vi "Main.vi"() -> ()   [LabVIEW 2018]
doc: "This VI simulates the acquisition of temperature, graphs the temperature, and notifies the user if the temperature is over the limit.\n\nThis VI is an exercise in the LabVIEW Basics II course and is used to experience property nodes."
panel:
  in  "Switch":bool
  in  "?":bool
  in  "Points to Acquire 8":i32=75 min=20 max=500
  in  "Points to Acquire 7":i32=75 min=20 max=500
  in  "Points to Acquire 6":i32=75 min=20 max=500
  in  "?":bool
  out "Remaining Time in Seconds":dbl
  in  "?":T1(tab)
  out "Temperature 2":T2(graph)
  out "5% Humidity":bool
  out "Temperature 9":T2(graph)
  out "5% Humidity":bool
  out "Temperature 10":T2(graph)
  out "5% Humidity":bool
  out "Temperature 11":T2(graph)
  out "5% Humidity":bool
  out "Weight Scale":dbl(knob) scale=0.0..10.0 scale format="%^#_6g"
  out "Weight Text Display":string
  in  "?":T3(tab)
  out "Temperature 3":T4(graph)
  out "7% Humidity":bool
  out "Temperature 6":T4(graph)
  out "7% Humidity":bool
  out "Temperature 7":T4(graph)
  out "7% Humidity":bool
  out "Temperature 8":T4(graph)
  out "7% Humidity":bool
  in  "Insert Cashew Nut Humidity Here":path
  in  "Insert Cashew Nut Weight":path
  in  "Heating Capacity":u32=400 min=50 max=2000 step=50
  out "Overload":bool
  in  "Points to Acquire 2":i32=75 min=20 max=500
  # "Drying Device"
  # "Roasting Device"
  # "Cashew Parameters"
  # "Device Parameters"
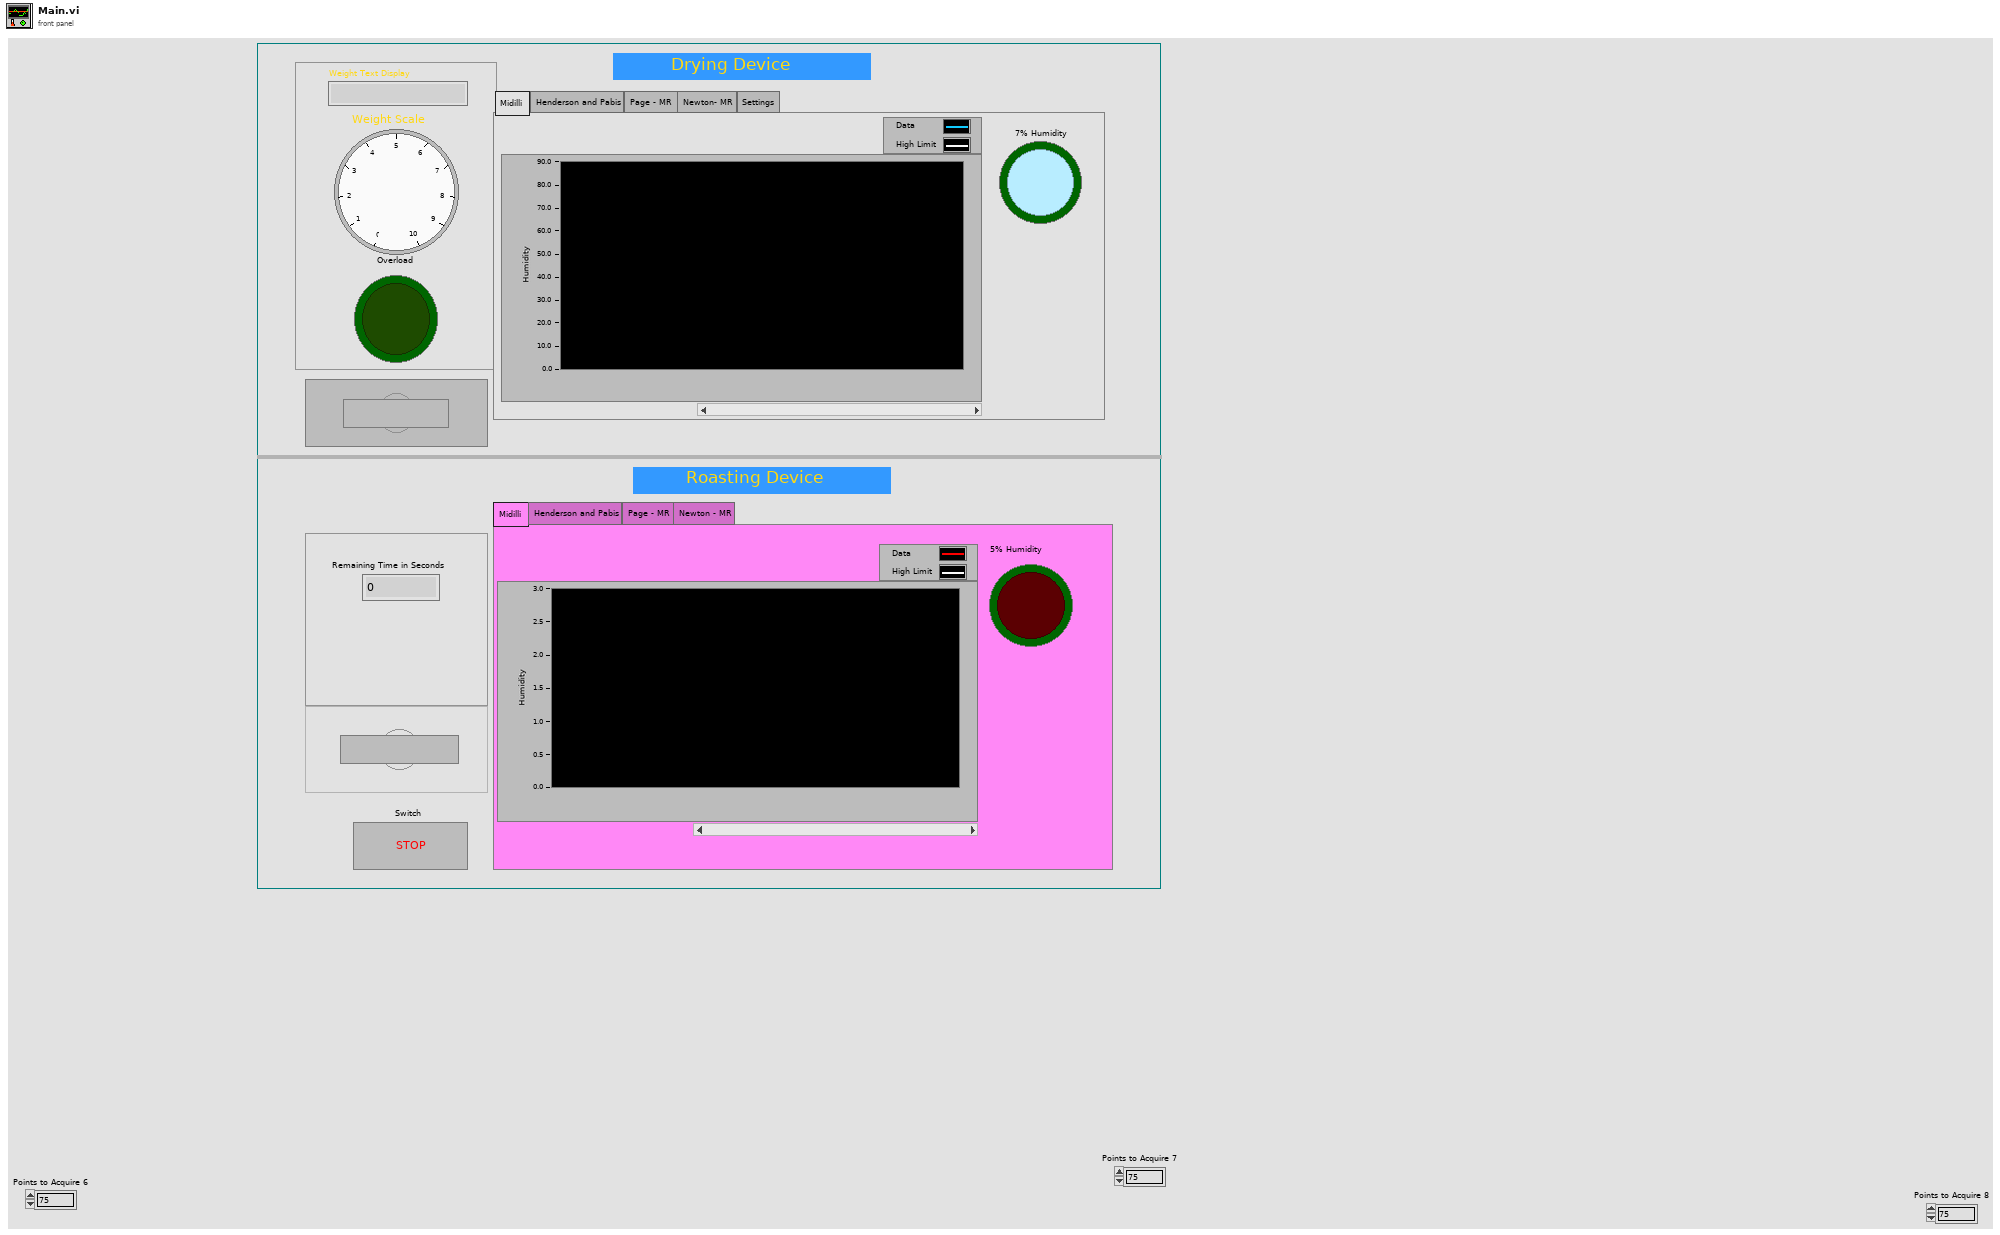
[diagram p1: front panel]
types:
  T1 = enum32{"Midilli", "Henderson and Pabis", "Page - MR", "Newton - MR"}
  T2 = cluster{"Temperature":dbl, "Temp High Limit 2":dbl}
  T3 = enum32{"Midilli", "Henderson and Pabis", "Page - MR ", "Newton- MR", "Settings"}
  T4 = cluster{"Humidity  High Limit":dbl, "Cashew Humidity":dbl}
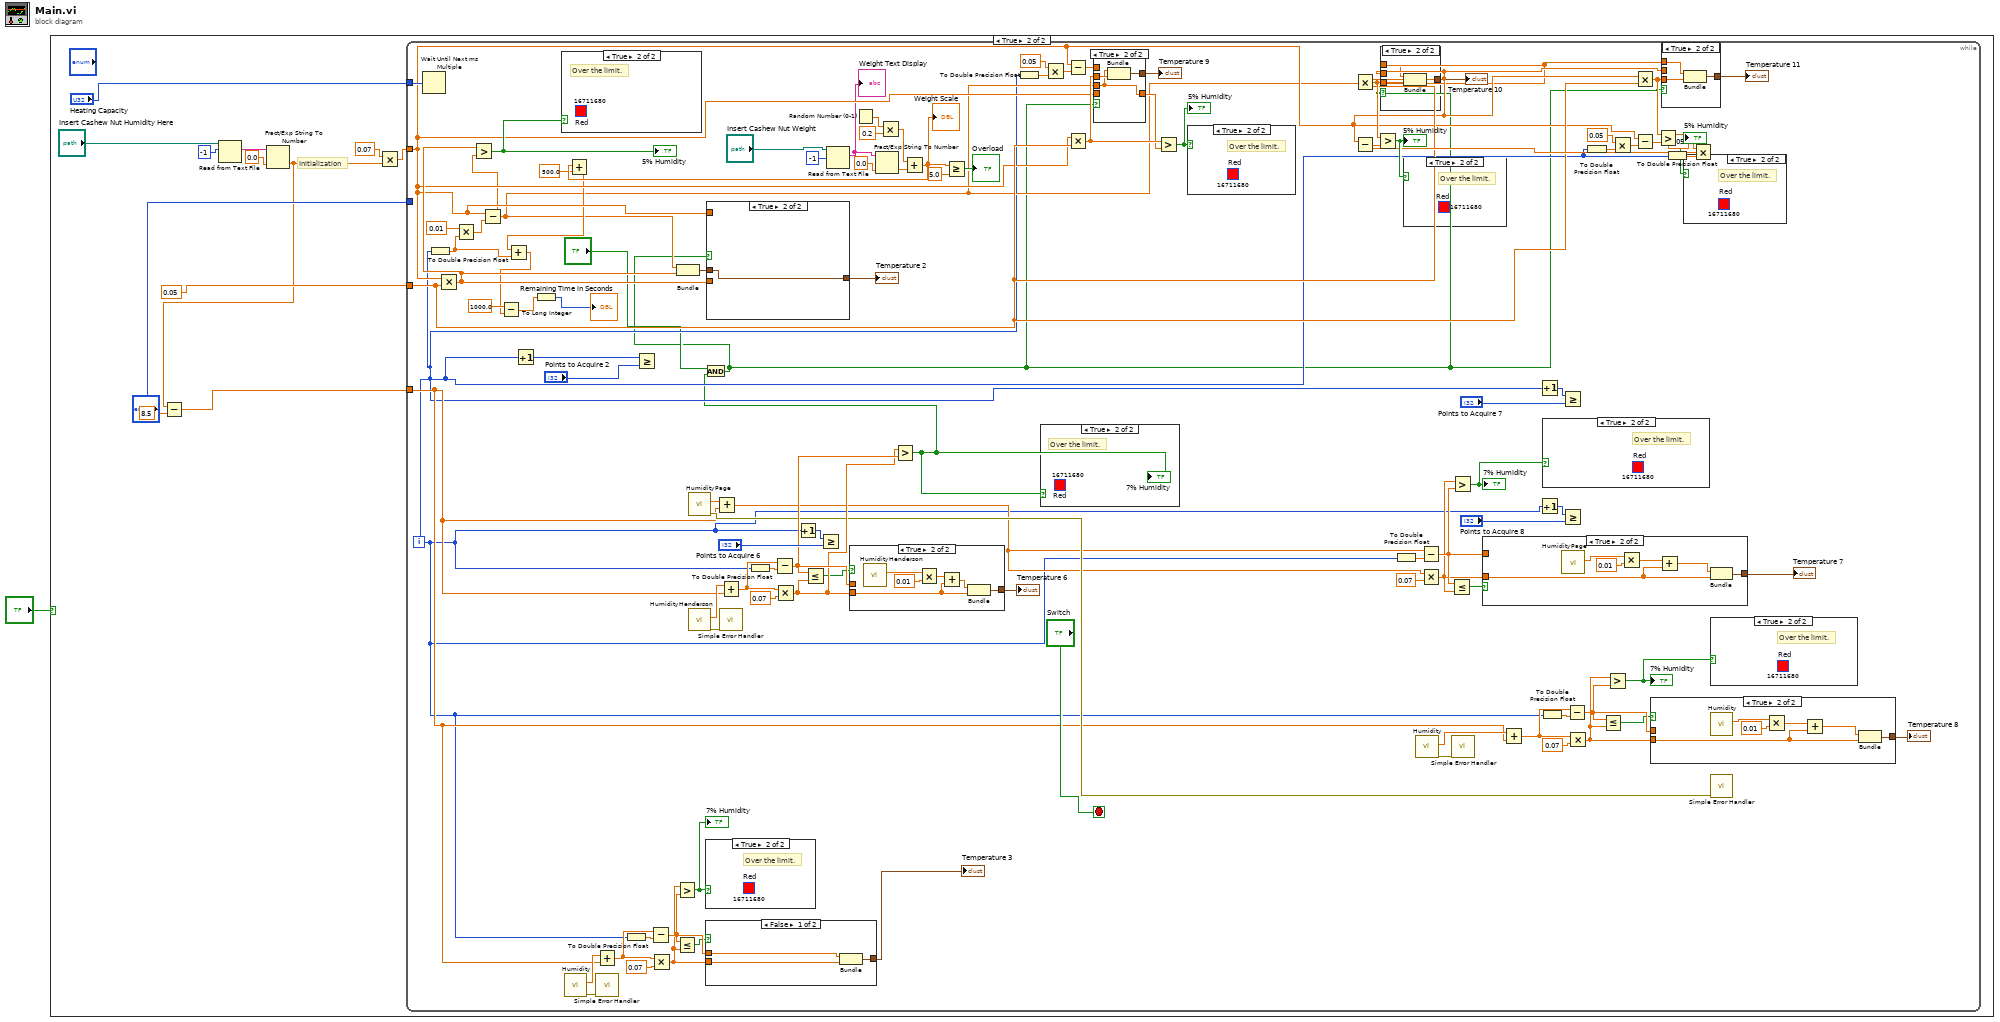
[diagram p0: block diagram]
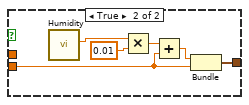
[diagram p3: hidden frame]
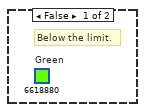
[diagram p4: hidden frame]
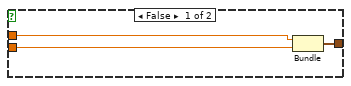
[diagram p5: hidden frame]
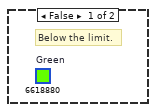
[diagram p6: hidden frame]
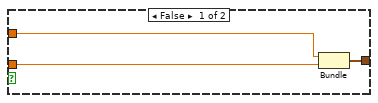
[diagram p7: hidden frame]
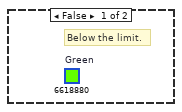
[diagram p8: hidden frame]
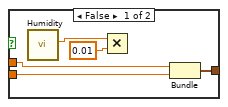
[diagram p9: hidden frame]
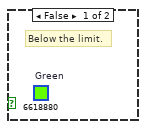
[diagram p10: hidden frame]
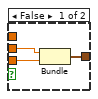
[diagram p11: hidden frame]
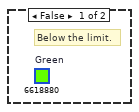
[diagram p12: hidden frame]
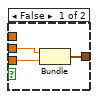
[diagram p13: hidden frame]
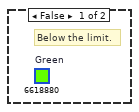
[diagram p14: hidden frame]
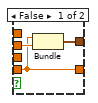
[diagram p15: hidden frame]
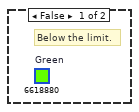
[diagram p16: hidden frame]
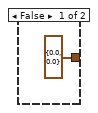
[diagram p17: hidden frame]
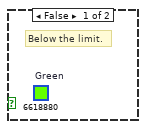
[diagram p18: hidden frame]
diagram:
  n1 = case shown="True" "?" {
    frame False {
    }
    frame True {
      # "Initialization"
      n2 = Read from Text File(file (use dialog)="Insert Cashew Nut Humidity Here", count=-1) -> (text=w11:string)  [unwired: 2 in, 3 out]
      n3 = Fract/Exp String To Number(string=w11, default (0 dbl)=0.0 ("default (0 DBL)")) -> (number=w4:dbl)  [unwired: 2 in, 1 out]
      n4 = Subtract(x=w4, y=8.5) -> (x-y=w2:dbl)
      n5 = Multiply(x=0.07, y=w4) -> (x*y=w8:dbl)
      n6 = while {
        tunnel: "Heating Capacity" -> [w114]
        tunnel: w8 -> [w86]
        tunnel: 0.05 ("x") -> [w87]
        tunnel: "?" -> [_]
        tunnel: w2 -> [w20]
        i -> [w19]
        stop <- "Switch" stop-if-true
        n7 = Wait Until Next ms Multiple(millisecond multiple=w114) -> ()  [unwired: 1 out]
        n8 = To Double Precision Float(number=w19) -> (double precision float=w74:dbl)
        n9 = Multiply(x=w86, y=w87) -> (x*y=w110:dbl)
        n10 = Multiply(x=0.01, y=w74) -> (x*y=w109:dbl)
        n11 = Subtract(x=w86, y=w109) -> (x-y=w66:dbl)
        n12 = Greater?(x=w110, y=w66) -> (0:w113:bool)
        "5% Humidity" <- w113
        n13 = Increment(x=w19) -> (x+1=w116:i32)
        n14 = case shown="True" w113 {
          frame False {
            (unwired) u32 6618880  # Green
            # "Below the limit."
          }
          frame True {
            (unwired) u32 16711680  # Red
            # "Over the limit."
          }
        }
        n15 = call "Humidity.vi"() -> ("error out"=w30:errorcluster, "Cashew Humidity"=w27:dbl)  [unwired: 10 in]
        n16 = Add(x=w27, y=w20) -> (x+y=w28:dbl)
        n17 = call <vilib>:"Simple Error Handler.vi"("error in (no error)"=w30) -> ()  [unwired: 4 in, 5 out]
        n18 = To Double Precision Float(number=w19) -> (double precision float=w24:dbl)
        n19 = Greater Or Equal?(x=w116, y="Points to Acquire 2") -> ()  [unwired: 1 out]
        n20 = Subtract(x=w28, y=w24) -> (x-y=w23:dbl)
        n21 = Multiply(x=w28, y=0.07) -> (x*y=w22:dbl)
        n22 = Greater?(x=w22, y=w23) -> (0:w25:bool)
        "7% Humidity" <- w25
        n23 = Less Or Equal?(x=w23, y=w22) -> (x <= y?=w21:bool)
        n24 = Bundle(w66, w110) -> (w15:cluster{dbl, dbl})  [unwired: 1 out]
        n25 = call "HumidityPage.vi"() -> ("error out"=w54:errorcluster, "Cashew Humidity"=w51:dbl)  [unwired: 10 in]
        n26 = call "HumidityHenderson.vi"() -> ("error out"=w65:errorcluster, "Cashew Humidity"=w63:dbl)  [unwired: 10 in]
        n27 = case shown="True" w25 {
          frame False {
            (unwired) u32 6618880  # Green
            # "Below the limit."
          }
          frame True {
            (unwired) u32 16711680  # Red
            # "Over the limit."
          }
        }
        n28 = case shown="False" w21 {
          tunnel: [w119 w125] -> w26
          tunnel: w23 -> [w117 _]
          tunnel: w22 -> [w118 w121]
          frame False {
            n29 = Bundle(w117, w118) -> (w119:cluster{dbl, dbl})  [unwired: 1 out]
          }
          frame True {
            n30 = call "Humidity.vi"() -> ("Cashew Humidity"=w124:dbl)  [unwired: 10 in, 1 out]
            n31 = Multiply(x=w124, y=0.01) -> (x*y=w122:dbl)
            n32 = Add(x=w122, y=w121) -> (x+y=w120:dbl)
            n33 = Bundle(w120, w121) -> (w125:cluster{dbl, dbl})  [unwired: 1 out]
          }
        }
        "Temperature 3" <- w26
        n34 = Add(x=w51, y=w20) -> (x+y=w52:dbl)
        n35 = Add(x=w63, y=w20) -> (x+y=w62:dbl)
        n36 = call <vilib>:"Simple Error Handler.vi"("error in (no error)"=w65) -> ()  [unwired: 4 in, 5 out]
        n37 = To Double Precision Float(number=w19) -> (double precision float=w58:dbl)
        n38 = Subtract(x=w62, y=w58) -> (x-y=w57:dbl)
        n39 = Multiply(x=w62, y=0.07) -> (x*y=w56:dbl)
        n40 = Increment(x=w19) -> (x+1=w60:i32)
        n41 = Less Or Equal?(x=w57, y=w56) -> (x <= y?=w55:bool)
        n42 = Greater Or Equal?(x=w60, y="Points to Acquire 6") -> ()  [unwired: 1 out]
        n43 = Read from Text File(file (use dialog)="Insert Cashew Nut Weight", count=-1) -> (text=w75:string)  [unwired: 2 in, 3 out]
        "Weight Text Display" <- w75
        n44 = case shown="True" w55 {
          tunnel: [w148 w154] -> w61
          tunnel: w57 -> [w147 _]
          tunnel: w56 -> [w146 w150]
          frame False {
            n45 = call "Humidity.vi"() -> ("Cashew Humidity"=w145:dbl)  [unwired: 10 in, 1 out]
            n46 = Multiply(x=w145, y=0.01) -> ()  [unwired: 1 out]
            n47 = Bundle(w147, w146) -> (w148:cluster{dbl, dbl})  [unwired: 1 out]
          }
          frame True {
            n48 = call "HumidityHenderson.vi"() -> ("Cashew Humidity"=w152:dbl)  [unwired: 10 in, 1 out]
            n49 = Multiply(x=w152, y=0.01) -> (x*y=w151:dbl)
            n50 = Add(x=w151, y=w150) -> (x+y=w149:dbl)
            n51 = Bundle(w149, w150) -> (w154:cluster{dbl, dbl})  [unwired: 1 out]
          }
        }
        "Temperature 6" <- w61
        n52 = Random Number (0-1)() -> (number: 0 to 1=w79:dbl)
        n53 = Fract/Exp String To Number(string=w75, default (0 dbl)=0.0 ("default (0 DBL)")) -> (number=w78:dbl)  [unwired: 2 in, 1 out]
        n54 = Multiply(x=w79, y=0.2) -> (x*y=w77:dbl)
        n55 = Greater?(x=w56, y=w57) -> (0:w16:bool)
        "7% Humidity" <- w16
        n56 = And(x="?", y=w16) -> (x .and. y?=w17:bool)
        n57 = case shown="True" w17 {
          tunnel: [cluster{dbl, dbl} {0.0, 0.0} w174] -> w14
          tunnel: w110 -> [_ _]
          tunnel: w86 -> [_ _]
          tunnel: w15 -> [_ w174]
          frame False {
          }
          frame True {
          }
        }
        "Temperature 2" <- w14
        n58 = Add(x=w77, y=w78) -> (x+y=w72:dbl)
        "Weight Scale" <- w72
        n59 = Add(x=w72, y=500.0) -> (x+y=w70:dbl)
        n60 = Add(x=w70, y=w74) -> (x+y=w73:dbl)
        n61 = Subtract(x=1000.0, y=w73) -> (x-y=w69:dbl)
        n62 = To Long Integer(number=w69) -> (32bit integer=→"Remaining Time in Seconds":i32)
        n63 = Greater Or Equal?(x=w72, y=5.0) -> (x >= y?=→"Overload":bool)
        n64 = To Double Precision Float(number=w19) -> (double precision float=w106:dbl)
        n65 = case shown="True" w16 {
          frame False {
            (unwired) u32 6618880  # Green
            # "Below the limit."
          }
          frame True {
            (unwired) u32 16711680  # Red
            # "Over the limit."
          }
        }
        n66 = Multiply(x=0.05, y=w106) -> (x*y=w103:dbl)
        n67 = Subtract(x=w86, y=w103) -> (x-y=w102:dbl)
        n68 = Multiply(x=w86, y=w87) -> (x*y=w104:dbl)
        n69 = case shown="True" w17 {
          tunnel: [w168 w172] -> w108
          tunnel: w104 -> [w169 w171]
          tunnel: w102 -> [_ _]
          tunnel: w86 -> [w167 _]
          tunnel: w66 -> [_ w170]
          tunnel: [w167 w170] -> w101
          frame False {
            n70 = Bundle(w167, w169) -> (w168:cluster{dbl, dbl})  [unwired: 1 out]
          }
          frame True {
            n71 = Bundle(w170, w171) -> (w172:cluster{dbl, dbl})  [unwired: 1 out]
          }
        }
        "Temperature 9" <- w108
        n72 = Greater?(x=w104, y=w101) -> (0:w107:bool)
        "5% Humidity" <- w107
        n73 = case shown="True" w107 {
          frame False {
            (unwired) u32 6618880  # Green
            # "Below the limit."
          }
          frame True {
            (unwired) u32 16711680  # Red
            # "Over the limit."
          }
        }
        n74 = Multiply(x=w86, y=w87) -> (x*y=w96:dbl)
        n75 = case shown="True" w17 {
          tunnel: [w162 w166] -> w100
          tunnel: w96 -> [w163 w165]
          tunnel: w66 -> [_ w164]
          tunnel: w86 -> [w161 _]
          frame False {
            n76 = Bundle(w161, w163) -> (w162:cluster{dbl, dbl})  [unwired: 1 out]
          }
          frame True {
            n77 = Bundle(w164, w165) -> (w166:cluster{dbl, dbl})  [unwired: 1 out]
          }
        }
        "Temperature 10" <- w100
        n78 = To Double Precision Float(number=w19) -> (double precision float=w47:dbl)
        n79 = call "Humidity.vi"() -> ("error out"=w42:errorcluster, "Cashew Humidity"=w40:dbl)  [unwired: 10 in]
        n80 = Subtract(x=w52, y=w47) -> (x-y=w46:dbl)
        n81 = Multiply(x=w52, y=0.07) -> (x*y=w45:dbl)
        n82 = Less Or Equal?(x=w46, y=w45) -> (x <= y?=w44:bool)
        n83 = Greater?(x=w45, y=w46) -> (0:w43:bool)
        "7% Humidity" <- w43
        n84 = call <vilib>:"Simple Error Handler.vi"("error in (no error)"=w42) -> ()  [unwired: 4 in, 5 out]
        n85 = case shown="True" w44 {
          tunnel: [w137 w143] -> w50
          tunnel: w46 -> [w136 _]
          tunnel: w45 -> [w135 w139]
          frame False {
            n86 = Bundle(w136, w135) -> (w137:cluster{dbl, dbl})  [unwired: 1 out]
          }
          frame True {
            n87 = call "HumidityPage.vi"() -> ("Cashew Humidity"=w141:dbl)  [unwired: 10 in, 1 out]
            n88 = Multiply(x=w141, y=0.01) -> (x*y=w140:dbl)
            n89 = Add(x=w140, y=w139) -> (x+y=w138:dbl)
            n90 = Bundle(w138, w139) -> (w143:cluster{dbl, dbl})  [unwired: 1 out]
          }
        }
        "Temperature 7" <- w50
        n91 = Add(x=w40, y=w20) -> (x+y=w39:dbl)
        n92 = Increment(x=w19) -> (x+1=w49:i32)
        n93 = Increment(x=w19) -> (x+1=w37:i32)
        n94 = To Double Precision Float(number=w19) -> (double precision float=w35:dbl)
        n95 = case shown="True" w43 {
          frame False {
            (unwired) u32 6618880  # Green
            # "Below the limit."
          }
          frame True {
            (unwired) u32 16711680  # Red
            # "Over the limit."
          }
        }
        n96 = Greater Or Equal?(x=w49, y="Points to Acquire 7") -> ()  [unwired: 1 out]
        n97 = Greater Or Equal?(x=w37, y="Points to Acquire 8") -> ()  [unwired: 1 out]
        n98 = Subtract(x=w39, y=w35) -> (x-y=w34:dbl)
        n99 = Multiply(x=w39, y=0.07) -> (x*y=w33:dbl)
        n100 = To Double Precision Float(number=w19) -> (double precision float=w91:dbl)
        n101 = Less Or Equal?(x=w34, y=w33) -> (x <= y?=w32:bool)
        n102 = Greater?(x=w33, y=w34) -> (0:w31:bool)
        "7% Humidity" <- w31
        n103 = Multiply(x=0.05, y=w91) -> (x*y=w89:dbl)
        n104 = Multiply(x=w86, y=w87) -> (x*y=w88:dbl)
        n105 = Subtract(x=w86, y=w89) -> (x-y=w67:dbl)
        n106 = case shown="True" w32 {
          tunnel: [w128 w134] -> w38
          tunnel: w34 -> [w127 _]
          tunnel: w33 -> [w126 w130]
          frame False {
            n107 = Bundle(w127, w126) -> (w128:cluster{dbl, dbl})  [unwired: 1 out]
          }
          frame True {
            n108 = call "Humidity.vi"() -> ("Cashew Humidity"=w132:dbl)  [unwired: 10 in, 1 out]
            n109 = Multiply(x=w132, y=0.01) -> (x*y=w131:dbl)
            n110 = Add(x=w131, y=w130) -> (x+y=w129:dbl)
            n111 = Bundle(w129, w130) -> (w134:cluster{dbl, dbl})  [unwired: 1 out]
          }
        }
        "Temperature 8" <- w38
        n112 = Greater?(x=w88, y=w67) -> (0:w92:bool)
        "5% Humidity" <- w92
        n113 = case shown="True" w17 {
          tunnel: [w156 w160] -> w93
          tunnel: w88 -> [w157 w159]
          tunnel: w66 -> [_ w158]
          tunnel: w86 -> [w155 _]
          frame False {
            n114 = Bundle(w155, w157) -> (w156:cluster{dbl, dbl})  [unwired: 1 out]
          }
          frame True {
            n115 = Bundle(w158, w159) -> (w160:cluster{dbl, dbl})  [unwired: 1 out]
          }
        }
        "Temperature 11" <- w93
        n116 = To Double Precision Float(number=w19) -> (double precision float=w98:dbl)
        n117 = case shown="True" w92 {
          frame False {
            (unwired) u32 6618880  # Green
            # "Below the limit."
          }
          frame True {
            (unwired) u32 16711680  # Red
            # "Over the limit."
          }
        }
        n118 = Multiply(x=0.05, y=w98) -> (x*y=w95:dbl)
        n119 = Subtract(x=w86, y=w95) -> (x-y=w94:dbl)
        n120 = Greater?(x=w96, y=w94) -> (0:w99:bool)
        "5% Humidity" <- w99
        n121 = case shown="True" w99 {
          frame False {
            (unwired) u32 6618880  # Green
            # "Below the limit."
          }
          frame True {
            (unwired) u32 16711680  # Red
            # "Over the limit."
          }
        }
        n122 = case shown="True" w31 {
          frame False {
            (unwired) u32 6618880  # Green
            # "Below the limit."
          }
          frame True {
            (unwired) u32 16711680  # Red
            # "Over the limit."
          }
        }
        n123 = call <vilib>:"Simple Error Handler.vi"("error in (no error)"=w54) -> ()  [unwired: 4 in, 5 out]
      }
    }
  }
